vi "Get LFO Test Specifications.vi"(8 "error in (no error)":errorcluster, 11 "configuration file path":path) -> (0 "error out":errorcluster, 1 "Test Specifications":dbl[](array[numeric]), 2 "key names":string[](array[string]))   [LabVIEW 2018]
uses:
  <vilib>/Utility/config.llb/Read Key (Double).vi
  <vilib>/Utility/config.llb/NI_LVConfig.lvlib
panel:
  out "section names":string[](array[string])
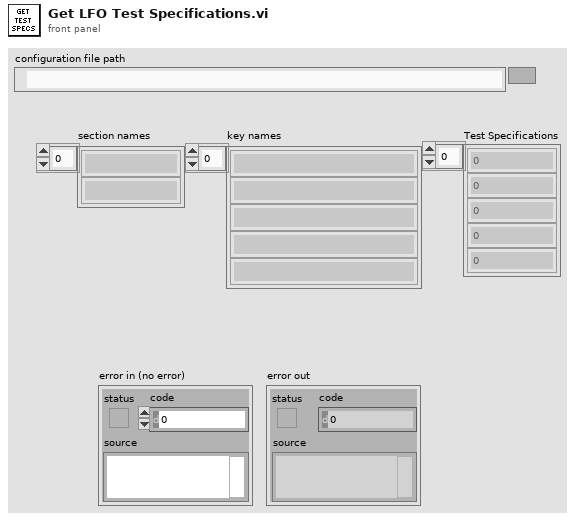
[diagram p1: front panel]
types:
  T1 = typedef "NI_LVConfig.lvlib/Config Data RefNum.ctl" = refnum<k1>
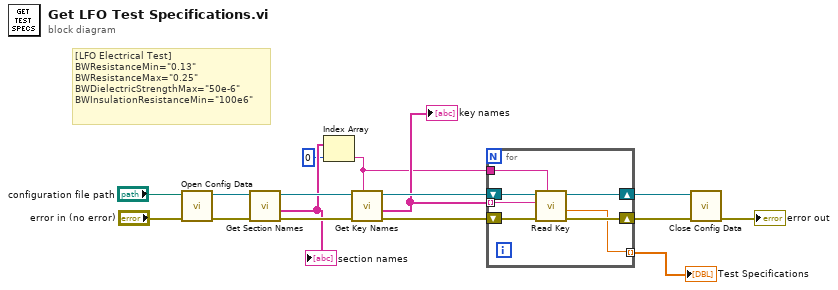
[diagram p0: block diagram]
diagram:
  # "[LFO Electrical Test]\nBWResistanceMin=\"0.13\"\nBWResistanceMax=\"0.25\"\nBWDielectricStrengthMax=\"50e-6\"\nBWInsulationResistanceMin=\"100e6\""
  n1 = call <vilib>:"Open Config Data.vi"("error in (no error)"="error in (no error)", "configuration file path"="configuration file path") -> ("error out"=w14:errorcluster, "refnum"=w12:T1)  [unwired: 7 in, 1 out]
  n2 = call <vilib>:"Get Section Names.vi"("error in (no error)"=w14, "refnum"=w12) -> ("error out"=w13:errorcluster, "section names"=w10:string[], "refnum out"=w11:T1)  [unwired: 7 in]
  "section names" <- w10
  n3 = Index Array(array=w10, index=0) -> (element=w3:string)
  n4 = call <vilib>:"Get Key Names.vi"("section"=w3, "error in (no error)"=w13, "refnum"=w11) -> ("error out"=w6:errorcluster, "key names"=w4:string[], "refnum out"=w8:T1)  [unwired: 5 in, 1 out]
  "key names" <- w4
  n5 = for {
    shift-right: [w22] -> w7
    shift-left: w8 -> [w23]
    shift-right: [w20] -> w5
    shift-left: w6 -> [w21]
    tunnel: w4 -> [w19] mode=indexing
    tunnel: w3 -> [w18]
    tunnel: [w17] -> w2 mode=indexing
    n6 = call-poly <vilib>:"Read Key.vi"("section"=w18, "error in (no error)"=w21, "key"=w19, "refnum"=w23) -> ("error out"=w20:errorcluster, "value"=w17:dbl, "refnum out"=w22:T1)  [unwired: 4 in, 1 out]
  }
  "Test Specifications" <- w2
  n7 = call <vilib>:"Close Config Data.vi"("error in (no error)"=w5, "refnum"=w7) -> ("error out"=→"error out":errorcluster)  [unwired: 8 in, 1 out]
